vi "QbusRef_FGV.vi"(7 "action":enum16{"Set", "Get"}(ring), 8 "error in (no error)":errorcluster, 11 "Qbus in":refnum<class "Qbus.lvclass">) -> (0 "error out":errorcluster, 3 "Qbus out":refnum<class "Qbus.lvclass">)   [LabVIEW 2017, in "Qbus.lvclass"]
uses:
  <vilib>/addons/Qbus/Qbus.lvclass
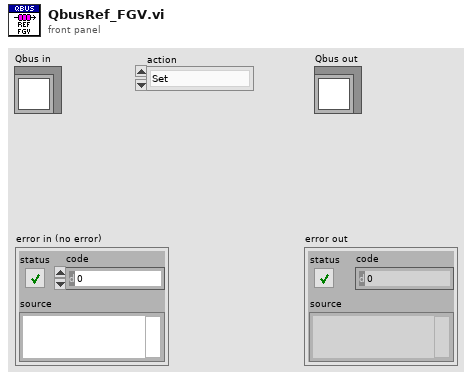
[diagram p1: front panel]
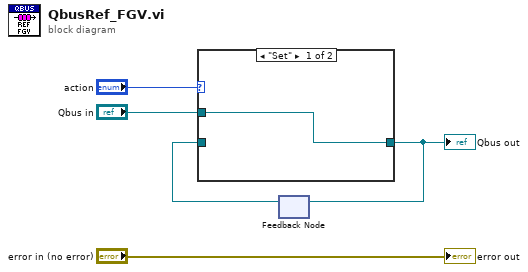
[diagram p0: block diagram]
diagram:
  n1 = feedback #1() -> (w1:refnum<class "Qbus.lvclass">)  [unwired: 1 in]
  n2 = case shown="\"Set\"" "action" {
    tunnel: "Qbus in" -> [w6 _]
    tunnel: [w6 w7] -> w2
    tunnel: w1 -> [_ w7]
    frame "Set" {
    }
    frame "Get", Default {
    }
  }
  "Qbus out" <- w2
  n3 = feedback-in #1(w2) -> ()
  "error out" <- "error in (no error)"
